vi "AH2700_Merge_Cluster.vi"(1 "AH 2700-Status":T1={"Units Display"=1, "Sample Switch"=0, "Frequency"=0.0, "V excitation"=0.0, "Capacity Graphic"=[], "Loss Graphic"=[], "Capacity"=0.0, "Loss"=0.0, "Bias "=0.0, " AVerage"=0.0} {"V excitation" format="%#_6f"; "Units Display" items=["nanosiemens"=1, "dissipation factor"=2, "kilohms"=3, "gigohms"=4, "loss vector (jpF)"=5]}, 2 "AH2700-Control":T2) -> (0 "AH 2700-Cluster":T3={"Units Display"=1, "Sample Switch"=0, "Frequency"=0.0, "V excitation"=0.0, "Capacity Graphic"=[], "Loss Graphic"=[], "Capacity"=0.0, "Loss"=0.0, "Update AH2500"=FALSE, "Bias "=0.0, " AVerage"=0.0} {"V excitation" format="%#_6f"; "Units Display" items=["nanosiemens"=1, "dissipation factor"=2, "kilohms"=3, "gigohms"=4, "loss vector (jpF)"=5]})   [LabVIEW 2019]
uses:
  AH2700/AH2700-Cluster.ctl
  AH2700/AH2700-Control.ctl
  AH2700/AH2700-Status.ctl
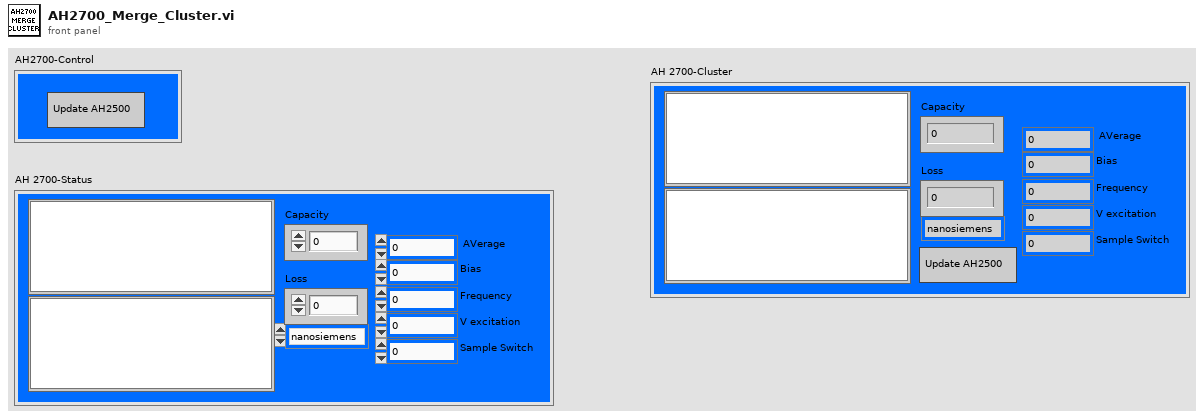
[diagram p1: front panel]
types:
  T1 = typedef "AH2700-Status.ctl" = cluster{"Units Display":i32, "Sample Switch":i32, "Frequency":dbl, "V excitation":dbl, "Capacity Graphic":dbl[][], "Loss Graphic":dbl[][], "Capacity":dbl, "Loss":dbl, "Bias ":dbl, " AVerage":dbl}
  T2 = typedef "AH2700-Control.ctl" = cluster{"Update AH2500":bool}
  T3 = typedef "AH2700-Cluster.ctl" = cluster{"Units Display":i32, "Sample Switch":i32, "Frequency":dbl, "V excitation":dbl, "Capacity Graphic":dbl[][], "Loss Graphic":dbl[][], "Capacity":dbl, "Loss":dbl, "Update AH2500":bool, "Bias ":dbl, " AVerage":dbl}
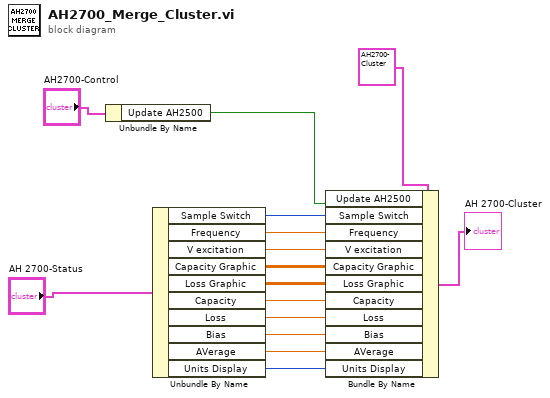
[diagram p0: block diagram]
diagram:
  n1 = Unbundle By Name("AH2700-Control") -> ("Update AH2500"=w12:bool)
  n2 = Unbundle By Name("AH 2700-Status") -> ("Sample Switch"=w10:i32, "Frequency"=w9:dbl, "V excitation"=w8:dbl, "Capacity Graphic"=w7:dbl[][], "Loss Graphic"=w6:dbl[][], "Capacity"=w5:dbl, "Loss"=w4:dbl, "Bias"=w3:dbl, "AVerage"=w2:dbl, "Units Display"=w1:i32)
  n3 = Bundle By Name(cluster=T3 {"Units Display"=1, "Sample Switch"=0, "Frequency"=0.0, "V excitation"=0.0, "Capacity Graphic"=[], "Loss Graphic"=[], "Capacity"=0.0, "Loss"=0.0, "Update AH2500"=FALSE, "Bias "=0.0, " AVerage"=0.0} ("AH 2700-Cluster"), "Update AH2500"=w12, "Sample Switch"=w10, "Frequency"=w9, "V excitation"=w8, "Capacity Graphic"=w7, "Loss Graphic"=w6, "Capacity"=w5, "Loss"=w4, "Bias"=w3, "AVerage"=w2, "Units Display"=w1) -> (→"AH 2700-Cluster":T3)
